vi "Initialize.vi"(8 "error in (no error)":errorcluster, 9 "PPLs Folder Path":path, 10 "INI File Path":path, 11 "Name":string) -> (0 "error out":errorcluster, 3 "Thermal Camera out":refnum<class "Thermal Camera.lvclass">)   [LabVIEW 2018, in "Thermal Camera.lvlib" / "Thermal Camera.lvclass"]
uses:
  Thermal Camera.lvclass
  Thermal Camera.lvclass/Thermal Camera.ctl
  PPLs/Configuration/Configuration.lvlibp/Configuration.lvclass
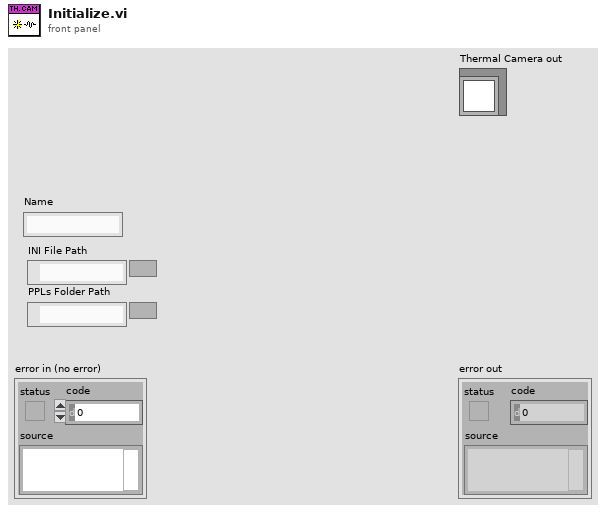
[diagram p1: front panel]
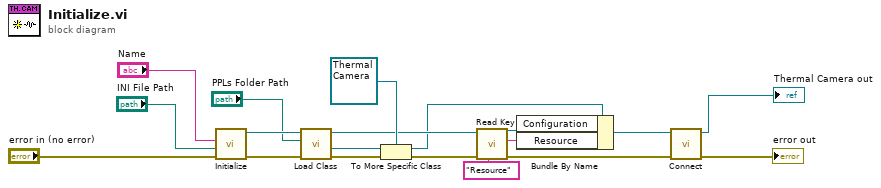
[diagram p0: block diagram]
diagram:
  n1 = call "Initialize.vi"("error in"="error in (no error)", "INI File Path"="INI File Path", "Device"="Name") -> ("error out"=w16:errorcluster, "Configuration out"=w15:refnum<class "Configuration.lvclass">)  [unwired: 7 in]
  n2 = call "Load Class.vi"("error in"=w16, "PPLs Folder Path"="PPLs Folder Path", "Configuration in"=w15) -> ("error out"=w13:errorcluster, "Class out"=w12:refnum<class>, "Configuration out"=w9:refnum<class "Configuration.lvclass">)  [unwired: 6 in]
  n3 = To More Specific Class(target class=refnum<class "Thermal Camera.lvclass"> refnum ("Thermal Camera.lvlib:Thermal Camera.lvclass"), reference=w12, error in=w13) -> (specific class reference=w7:refnum<class "Thermal Camera.lvclass">, error out=w10:errorcluster)
  n4 = call "Read Key.vi"("Key:"="Resource", "error in"=w10, "Configuration in"=w9) -> ("error out"=w3:errorcluster, "Value"=w6:string, "Configuration out"=w5:refnum<class "Configuration.lvclass">)  [unwired: 6 in]
  n5 = Bundle By Name(cluster=w7, "Configuration"=w5, "Resource"=w6) -> (w4:refnum<class "Thermal Camera.lvclass">)
  n6 = call-dynamic "Connect.vi"("error in (no error)"=w3, "Thermal Camera in"=w4) -> ("error out"=→"error out":errorcluster, "Thermal Camera out"=→"Thermal Camera out":refnum<class "Thermal Camera.lvclass">)  [unwired: 8 in]
